vi "Set Merge-Delegate.vi"(8 "error in (no error)":errorcluster, 10 "Merge-Delegate":refnum<class "Merge-Delegate.lvclass">, 11 "Git Implementation in":refnum<class "Git Implementation.lvclass">) -> (0 "error out":errorcluster, 3 "Git Implementation out":refnum<class "Git Implementation.lvclass">)   [LabVIEW 2017, in "Git-LabVIEW.lvlib" / "Git Implementation.lvclass"]
uses:
  Git Implementation.lvclass
  Merge Operations/Interface/Merge-Delegate.lvclass
  Git Implementation.lvclass/Git Implementation.ctl
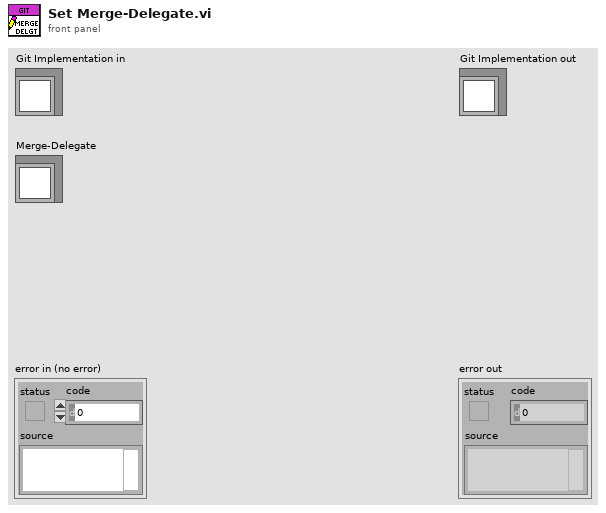
[diagram p1: front panel]
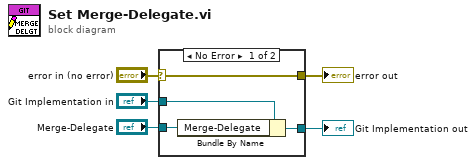
[diagram p0: block diagram]
diagram:
  n1 = case shown="No Error" "error in (no error)" {
    selector: "error in (no error)" -> [w9 w10]
    tunnel: [w9 w10] -> w4
    tunnel: [w7 w11] -> w2
    tunnel: "Git Implementation in" -> [w8 w11]
    tunnel: "Merge-Delegate" -> [w6 _]
    frame No Error {
      n2 = Bundle By Name(cluster=w8, "Merge-Delegate"=w6) -> (w7:refnum<class "Git Implementation.lvclass">)
    }
    frame Error {
    }
  }
  "error out" <- w4
  "Git Implementation out" <- w2
